vi "Generate .avi filenames.vi"(8 "Camera 2?":bool, 9 "Spark counter":i32, 10 "AVI File Path 2":path=path "C:/Users/CeNTREX/Documents/Electrostatic lens data/Looking for sparks/Videos/ ", 11 "AVI File Path":path=path "C:/Users/CeNTREX/Documents/Electrostatic lens data/Looking for sparks/Videos/ ") -> (2 "AVI path 2":path, 3 "AVI path 1":path)   [LabVIEW 2018]
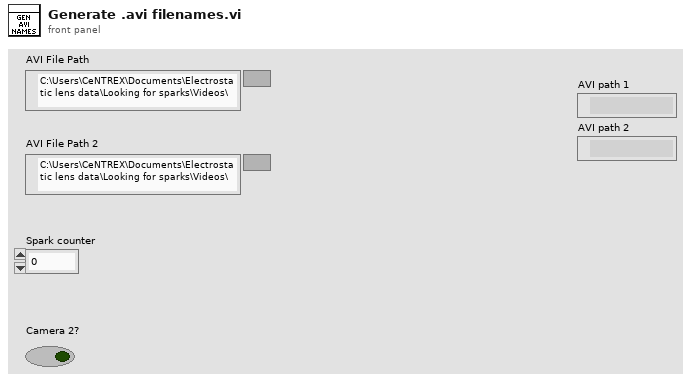
[diagram p1: front panel]
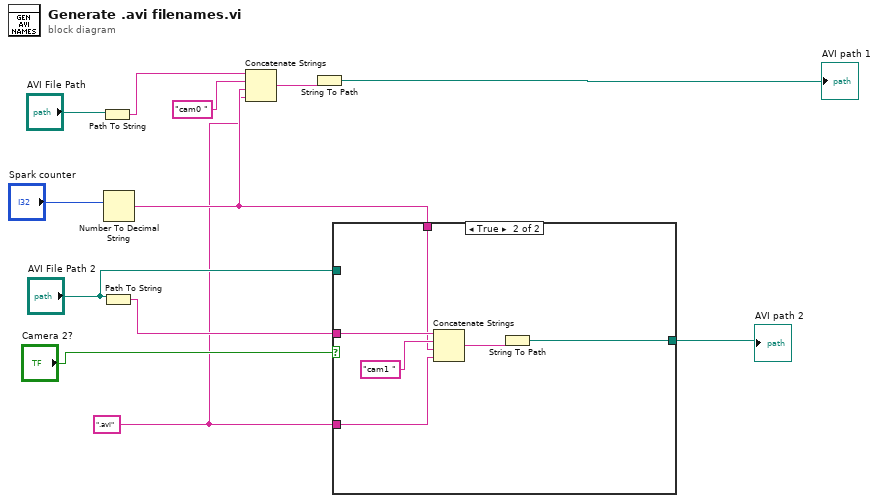
[diagram p0: block diagram]
diagram:
  w1 = ".avi"
  n1 = Path To String(path="AVI File Path") -> (string=w10:string)
  n2 = Path To String(path="AVI File Path 2") -> (string=w6:string)
  n3 = Number To Decimal String(number="Spark counter") -> (decimal integer string=w5:string)  [unwired: 1 in]
  n4 = Concatenate Strings(w10, "cam0 ", w5, w1) -> (w9:string)
  n5 = String To Path(string=w9) -> (path=→"AVI path 1":path)
  n6 = case shown="True" "Camera 2?" {
    tunnel: w6 -> [_ w18]
    tunnel: w5 -> [_ w17]
    tunnel: [w13 w15] -> w4
    tunnel: "AVI File Path 2" -> [w13 _]
    tunnel: w1 -> [_ w14]
    frame False {
    }
    frame True {
      n7 = Concatenate Strings(w18, "cam1 ", w17, w14) -> (w16:string)
      n8 = String To Path(string=w16) -> (path=w15:path)
    }
  }
  "AVI path 2" <- w4
